vi "WeDo-PyBD.vi"() -> ()   [LabVIEW 2016]
uses:
  VIs/uPythonX/uPythonX.xctl
panel:
  in  "Tab Control":T1(tab)=enum."Line Follow"
  in  "WeDo Sniffing Code":T2(xcontrol)={"VISA Refnum in"="ASRL23::INSTR", "Python Code"="import machine, utime\n\nuart = machine.UART(3)\nuart.init(baudrate=2400, bits=8, parity=None, stop=1)\n\nutime.sleep_ms(1000)\n\nstring = ''\nsize = 1\nwhile True:\n     print(uart.read(uart.any()))\n     utime.sleep_ms(300)\n     size = uart.any()\n\nstring"}
  in  "WeDo":T2(xcontrol)={"VISA Refnum in"="ASRL12::INSTR", "Python Code"="import machine, utime, gc\n\nuart = machine.UART(1)\n\ndef send_value(uart,data):\n     value = (data & 0xFF)\n     payload = bytes([0xC0, value, 0xFF ^ 0xC0 ^ value])\n     uart.write(payload)\n\ndef initLPF2(uart):\n     tx = machine.Pin('P1', machine.Pin.OUT)\n     rx = machine.Pin('P0', machine.Pin.IN)\n     tx.value(0)\n     utime.sleep_ms(500)\n     tx.value(1)\n     uart.init(baudrate=2400, bits=8, parity=None, stop=1)\n     uart.write(b'\\x00')\n     uart.write(b'\\x40\\x23\\x9C')\n     uart.write(b'\\x49\\x02\\x01\\xB5')\n     uart.write(b'\\x52\\x00\\xC2\\x01\\x00\\x6E')\n     uart.write(b'\\x5F\\x00\\x00\\x00\\x02\\x00\\x00\\x00\\x02\\xA0')\n     uart.write(b'\\x9A\\x00\\x4C\\x50\\x46\\x32\\x2D\\x43\\x41\\x4C\\x6E')\n     uart.write(b'\\x9A\\x01\\x00\\x00\\x00\\x00\\x00\\xC0\\x7F\\x44\\x9F')\n     uart.write(b'\\x9A\\x02\\x00\\x00\\x00\\x00\\x00\\x00\\xC8\\x42\\xED')\n     uart.write(b'\\x9A\\x03\\x00\\x00\\x00\\x00\\x00\\xC0\\x7F\\x44\\x9D')\n     uart.write(b'\\x92\\x04\\x52\\x41\\x57\\x00\\x2D')\n     uart.write(b'\\x8A\\x05\\x10\\x00\\x60')\n     uart.write(b'\\x92\\x80\\x03\\x01\\x03\\x00\\xEC')\n     utime.sleep_ms(5)\n     print(uart.read(uart.any()))\n     uart.write(b'\\xA1\\x00\\x4C\\x50\\x46\\x32\\x2D\\x43\\x4F\\x55\\x4E\\x54\\x00\\x00\\x00\\x00\\x00\\x00\\x58')\n     uart.write(b'\\x99\\x01\\x00\\x00\\x00\\x00\\x00\\x00\\xC8\\x42\\xED')\n     uart.write(b'\\x99\\x02\\x00\\x00\\x00\\x00\\x00\\x00\\xC8\\x42\\xEE')\n     uart.write(b'\\x99\\x03\\x00\\x00\\x00\\x00\\x00\\x00\\xC8\\x42\\xEF')\n     uart.write(b'\\x91\\x04\\x43\\x4E\\x54\\x00\\x33')\n     uart.write(b'\\x89\\x05\\x10\\x00\\x63')\n     uart.write(b'\\x91\\x80\\x01\\x02\\x04\\x00\\xE9')\n     utime.sleep_ms(5)\n     print(uart.read(uart.any()))\n     uart.write(b'\\xA0\\x00\\x4C\\x50\\x46\\x32\\x2D\\x44\\x45\\x54\\x45\\x43\\x54\\x00\\x00\\x00\\x00\\x00\\x1D')\n     uart.write(b'\\x98\\x01\\x00\\x00\\x00\\x00\\x00\\x00\\x20\\x41\\x07')\n     uart.write(b'\\x98\\x02\\x00\\x00\\x00\\x00\\x00\\x00\\xC8\\x42\\xEF')\n     uart.write(b'\\x98\\x03\\x00\\x00\\x00\\x00\\x00\\x00\\x20\\x41\\x05')\n     uart.write(b'\\x80\\x04\\x00\\x7B')\n     uart.write(b'\\x88\\x05\\x10\\x00\\x62')\n     uart.write(b'\\x90\\x80\\x01\\x00\\x03\\x00\\xED')\n     utime.sleep_ms(5)\n     print(uart.read(uart.any()))\n     uart.write(b'\\x04')  \n     # wait for ACK\n     starttime = utime.time()\n     currenttime = starttime\n     while (currenttime-starttime) < 2000:\n          utime.sleep_ms(5)\n          data = uart.read(uart.any())\n          if data.find(b'\\x04') >= 0:\n               print('Success')\n               currenttime = starttime+3000   # stop the loop\n          else:\n               currenttime = utime.time()\n     # pull pin low\n     uart.deinit()\n     tx = machine.Pin('P1', machine.Pin.OUT)\n     tx.value(0)\n     utime.sleep_ms(10)\n     #change baudrate\n     uart.init(baudrate=115200, bits=8, parity=None, stop=1)\n\n# loop from -10 to 10\ni=0\ninitLPF2(uart)\nwhile True:\n     gc.collect()\n     send_value(uart,i)\n     i += 1\n     if i > 10: i=-10\n     utime.sleep_ms(200)\n"}
  in  "LPF2Class":T2(xcontrol)={"VISA Refnum in"="ASRL12::INSTR", "Python Code"="import machine, utime, gc\n\nfrom pyb import LED\n\nred_led   = LED(1)\ngreen_led = LED(2)\nblue_led  = LED(3)\nir_led    = LED(4)\n\nclass LPF2(object):\n     def __init__(self, uartChannel, txPin, rxPin):\n          self.txPin = txPin\n          self.rxPin = rxPin\n          self.uart = machine.UART(uartChannel)\n          self.connected = False\n\n     def send_value(self,data):\n          value = (data & 0xFF)\n          payload = bytes([0xC0, value, 0xFF ^ 0xC0 ^ value])\n          size = self.uart.write(payload)\n          if not size: self.connected = False\n\n     def initialize(self):\n          self.tx = machine.Pin(self.txPin, machine.Pin.OUT)\n          self.rx = machine.Pin(self.rxPin, machine.Pin.IN)\n          self.tx.value(0)\n          utime.sleep_ms(500)\n          self.tx.value(1)\n          self.uart.init(baudrate=2400, bits=8, parity=None, stop=1)\n          self.uart.write(b'\\x00')\n          self.uart.write(b'\\x40\\x23\\x9C')\n          self.uart.write(b'\\x49\\x02\\x01\\xB5')\n          self.uart.write(b'\\x52\\x00\\xC2\\x01\\x00\\x6E')\n          self.uart.write(b'\\x5F\\x00\\x00\\x00\\x02\\x00\\x00\\x00\\x02\\xA0')\n          self.uart.write(b'\\x9A\\x00\\x4C\\x50\\x46\\x32\\x2D\\x43\\x41\\x4C\\x6E')\n          self.uart.write(b'\\x9A\\x01\\x00\\x00\\x00\\x00\\x00\\xC0\\x7F\\x44\\x9F')\n          self.uart.write(b'\\x9A\\x02\\x00\\x00\\x00\\x00\\x00\\x00\\xC8\\x42\\xED')\n          self.uart.write(b'\\x9A\\x03\\x00\\x00\\x00\\x00\\x00\\xC0\\x7F\\x44\\x9D')\n          self.uart.write(b'\\x92\\x04\\x52\\x41\\x57\\x00\\x2D')\n          self.uart.write(b'\\x8A\\x05\\x10\\x00\\x60')\n          self.uart.write(b'\\x92\\x80\\x03\\x01\\x03\\x00\\xEC')\n          utime.sleep_ms(5)\n          #  print(uart.read(uart.any()))\n          self.uart.write(b'\\xA1\\x00\\x4C\\x50\\x46\\x32\\x2D\\x43\\x4F\\x55\\x4E\\x54\\x00\\x00\\x00\\x00\\x00\\x00\\x58')\n          self.uart.write(b'\\x99\\x01\\x00\\x00\\x00\\x00\\x00\\x00\\xC8\\x42\\xED')\n          self.uart.write(b'\\x99\\x02\\x00\\x00\\x00\\x00\\x00\\x00\\xC8\\x42\\xEE')\n          self.uart.write(b'\\x99\\x03\\x00\\x00\\x00\\x00\\x00\\x00\\xC8\\x42\\xEF')\n          self.uart.write(b'\\x91\\x04\\x43\\x4E\\x54\\x00\\x33')\n          self.uart.write(b'\\x89\\x05\\x10\\x00\\x63')\n          self.uart.write(b'\\x91\\x80\\x01\\x02\\x04\\x00\\xE9')\n          utime.sleep_ms(5)\n          # print(uart.read(uart.any()))\n          self.uart.write(b'\\xA0\\x00\\x4C\\x50\\x46\\x32\\x2D\\x44\\x45\\x54\\x45\\x43\\x54\\x00\\x00\\x00\\x00\\x00\\x1D')\n          self.uart.write(b'\\x98\\x01\\x00\\x00\\x00\\x00\\x00\\x00\\x20\\x41\\x07')\n          self.uart.write(b'\\x98\\x02\\x00\\x00\\x00\\x00\\x00\\x00\\xC8\\x42\\xEF')\n          self.uart.write(b'\\x98\\x03\\x00\\x00\\x00\\x00\\x00\\x00\\x20\\x41\\x05')\n          self.uart.write(b'\\x80\\x04\\x00\\x7B')\n          self.uart.write(b'\\x88\\x05\\x10\\x00\\x62')\n          self.uart.write(b'\\x90\\x80\\x01\\x00\\x03\\x00\\xED')\n          utime.sleep_ms(5)\n          # print(uart.read(uart.any()))\n          self.uart.write(b'\\x04')  \n          # wait for ACK\n          starttime = utime.time()\n          currenttime = starttime\n          while (currenttime-starttime) < 2000:\n               utime.sleep_ms(5)\n               data = self.uart.read(self.uart.any())\n               if data.find(b'\\x04') >= 0:\n                    self.connected = True\n                    currenttime = starttime+3000   # stop the loop\n               else:\n                    currenttime = utime.time()\n          # pull pin low\n          self.uart.deinit()\n          self.tx = machine.Pin(self.txPin, machine.Pin.OUT)\n          self.tx.value(0)\n          utime.sleep_ms(10)\n          #change baudrate\n          self.uart.init(baudrate=115200, bits=8, parity=None, stop=1)"}
  in  "ToSpike":T2(xcontrol)={"VISA Refnum in"="ASRL12::INSTR", "Python Code"="import LPF2Class\n\n# loop from -10 to 10\ni=0\nred_led.on()\nlpf2 = LPF2Class.LPF2(1, 'P1', 'P0')    # OpenMV\nlpf2.initialize()\n\nwhile True:\n     if not lpf2.connected:\n          red_led.on()\n          utime.sleep(1)\n          lpf2.initialize()\n     else:\n          red_led.off()\n          while lpf2.connected:\n               gc.collect()\n               lpf2.send_value(i)\n               i += 1\n               # print(lpf2.connected)\n               if i > 10: i=-10\n               utime.sleep_ms(200)\n"}
  in  "ToSpike 2":T2(xcontrol)={"VISA Refnum in"="ASRL12::INSTR", "Python Code"="import LPF2Class\nimport sensor, image, time\n\nenable_lens_corr = False # turn on for straighter lines...\n\nsensor.reset()\nsensor.set_pixformat(sensor.RGB565) # grayscale is faster\nsensor.set_framesize(sensor.QQVGA)\nsensor.skip_frames(time = 2000)\n\nmin_degree = 0\nmax_degree = 179\n\n\nred_led.on()\nlpf2 = LPF2Class.LPF2(1, 'P1', 'P0')    # OpenMV\nlpf2.connected = True\n#lpf2.initialize()\n\nwhile True:\n     img = sensor.snapshot()\n     if enable_lens_corr: img.lens_corr(1.8) # for 2.8mm lens...\n          \n     if not lpf2.connected:\n          red_led.on()\n          utime.sleep(1)\n          lpf2.initialize()\n     else:\n          red_led.off()\n          while lpf2.connected:\n               gc.collect()\n               rawLines = img.find_lines(threshold = 1000, theta_margin = 25, rho_margin = 25)\n               averageAngle = 0\n               for line in rawLines:\n                    if (min_degree <= line.theta()) and (line.theta() <= max_degree):\n                         img.draw_line(line.line(), color = (255, 0, 0))\n                         averageAngle + = line.theta()\n               value = averageAngle / len(rawLines)\n\n               lpf2.send_value(value)\n               print(value)\n               utime.sleep_ms(200)\n"}
  in  "Spike":T2(xcontrol)={"VISA Refnum in"="ASRL73::INSTR", "Python Code"="import hub,utime\n\nhub.port.B.info()\n\n# if info comes back with None - then you have to restart the pybaord\n\nwhile True:\n     try:\n          value = hub.port.B.device.get()[0]\n          # print(value)\n          hub.display.show(str(value))\n          utime.sleep(0.2)\n     except:\n          utime.sleep(1)\n"}
  in  "WeDo 2":T2(xcontrol)={"VISA Refnum in"="ASRL23::INSTR", "Python Code"="import machine, utime, gc\n\ndef send_value(data):\n     value = (data & 0xFF)\n     payload = bytes([0xC0, value, 0xFF ^ 0xC0 ^ value])\n     uart.write(payload)\n\nimport machine, network, ubinascii, ujson, urequests\n\nWiFi = network.WLAN()\n\nmac = ubinascii.hexlify(network.WLAN().config(\"mac\"),\":\").decode()\nprint(\"MAC address: \" + mac)\n\ndef connect():\n     EN1 = machine.Pin(\"W23\", machine.Pin.OUT, value=1)  # set power high for USB power (500mA now allowed)\n     if not WiFi.isconnected():\n          print (\"Connecting ..\")\n          WiFi.active(True)\n          WiFi.connect(\"Chris's iPhone\",\"00lly4r4uryu\")\n          i=0\n          while i < 25 and not WiFi.isconnected():\n               utime.sleep_ms(200)\n               i=i+1\n          if WiFi.isconnected():\n               print (\"Connection succeeded\")\n          else:\n               print (\"Connection failed\")     \n\nconnect()\nprint (\"WiFi: \",WiFi.isconnected())\n\n# Info\nTag = \"admin.HiPeaks.temperature\"\nType = \"DOUBLE\"\nValue = \"0\"\nKey = \"0MasdJmBFsHePZqAtGn-_3xky4M8rxeNPjaSO4H5u9\"\n\nurlBase = \"https://api.systemlinkcloud.com/nitag/v2/tags/\"\nheaders = {\"Accept\":\"application/json\",\"x-ni-api-key\":Key}\n\nurlValue = urlBase + Tag + \"/values/current\"\n\ndef grab_value():\n#     value = {'value':'0'}\n     try:\n          value = urequests.get(urlValue,headers=headers).text\n     except:\n          pass\n\n     data = ujson.loads(value)\n     result = data.get(\"value\").get(\"value\")\n     return result\n\n# prepare WeDo\n\ntx = machine.Pin('Y9', machine.Pin.OUT)\nrx = machine.Pin('Y10', machine.Pin.IN)\ntx.value(0)\nutime.sleep_ms(500)\ntx.value(1)\n\nuart = machine.UART(3)\nuart.init(baudrate=2400, bits=8, parity=None, stop=1)\n\nuart.write(b'\\x00')\nuart.write(b'\\x40\\x23\\x9C')\nuart.write(b'\\x49\\x02\\x01\\xB5')\nuart.write(b'\\x52\\x00\\xC2\\x01\\x00\\x6E')\nuart.write(b'\\x5F\\x00\\x00\\x00\\x02\\x00\\x00\\x00\\x02\\xA0')\nuart.write(b'\\x9A\\x00\\x4C\\x50\\x46\\x32\\x2D\\x43\\x41\\x4C\\x6E')\nuart.write(b'\\x9A\\x01\\x00\\x00\\x00\\x00\\x00\\xC0\\x7F\\x44\\x9F')\nuart.write(b'\\x9A\\x02\\x00\\x00\\x00\\x00\\x00\\x00\\xC8\\x42\\xED')\nuart.write(b'\\x9A\\x03\\x00\\x00\\x00\\x00\\x00\\xC0\\x7F\\x44\\x9D')\nuart.write(b'\\x92\\x04\\x52\\x41\\x57\\x00\\x2D')\nuart.write(b'\\x8A\\x05\\x10\\x00\\x60')\nuart.write(b'\\x92\\x80\\x03\\x01\\x03\\x00\\xEC')\nutime.sleep_ms(5)\nprint(uart.read(uart.any()))\nuart.write(b'\\xA1\\x00\\x4C\\x50\\x46\\x32\\x2D\\x43\\x4F\\x55\\x4E\\x54\\x00\\x00\\x00\\x00\\x00\\x00\\x58')\nuart.write(b'\\x99\\x01\\x00\\x00\\x00\\x00\\x00\\x00\\xC8\\x42\\xED')\nuart.write(b'\\x99\\x02\\x00\\x00\\x00\\x00\\x00\\x00\\xC8\\x42\\xEE')\nuart.write(b'\\x99\\x03\\x00\\x00\\x00\\x00\\x00\\x00\\xC8\\x42\\xEF')\nuart.write(b'\\x91\\x04\\x43\\x4E\\x54\\x00\\x33')\nuart.write(b'\\x89\\x05\\x10\\x00\\x63')\nuart.write(b'\\x91\\x80\\x01\\x02\\x04\\x00\\xE9')\nutime.sleep_ms(5)\nprint(uart.read(uart.any()))\nuart.write(b'\\xA0\\x00\\x4C\\x50\\x46\\x32\\x2D\\x44\\x45\\x54\\x45\\x43\\x54\\x00\\x00\\x00\\x00\\x00\\x1D')\nuart.write(b'\\x98\\x01\\x00\\x00\\x00\\x00\\x00\\x00\\x20\\x41\\x07')\nuart.write(b'\\x98\\x02\\x00\\x00\\x00\\x00\\x00\\x00\\xC8\\x42\\xEF')\nuart.write(b'\\x98\\x03\\x00\\x00\\x00\\x00\\x00\\x00\\x20\\x41\\x05')\nuart.write(b'\\x80\\x04\\x00\\x7B')\nuart.write(b'\\x88\\x05\\x10\\x00\\x62')\nuart.write(b'\\x90\\x80\\x01\\x00\\x03\\x00\\xED')\nutime.sleep_ms(5)\nprint(uart.read(uart.any()))\nuart.write(b'\\x04')\n\n# wait for ACK\nstarttime = utime.time()\ncurrenttime = starttime\n\nwhile (currenttime-starttime) < 2000:\n     utime.sleep_ms(5)\n     data = uart.read(uart.any())\n     if data.find(b'\\x04') >= 0:\n          print('Success')\n          currenttime = starttime+3000   # stop the loop\n     else:\n          currenttime = utime.time()\n\n# pull pin low\nuart.deinit()\ntx = machine.Pin('Y9', machine.Pin.OUT)\ntx.value(0)\nutime.sleep_ms(10)\n\n#change baudrate\n\nuart.init(baudrate=115200, bits=8, parity=None, stop=1)\n\n# loop from -10 to 10\ni=0\n\nwhile True:\n     gc.collect()\n     data = grab_value()\n     send_value(data)\n     i += 1\n     if i > 10: i=-10\n     utime.sleep_ms(200)\n"}
  in  "Test":T2(xcontrol)={"VISA Refnum in"="ASRL23::INSTR", "Python Code"="import machine, utime\n\n\nuart = machine.UART(6)\nuart.init(baudrate=2400, bits=8, parity=None, stop=1)\n\nuart.write(b'\\x40\\x23\\x9C')\nutime.sleep_ms(1000)\nuart.read(uart.any())"}
  in  "Hub":T2(xcontrol)={"VISA Refnum in"="ASRL24::INSTR", "Python Code"="import hub,utime\n\n# no idea how to read a sesnor value on flipper - how do I read the \n#accelerometer as well?\n\nhub.button.left.is_pressed()\n\nhub.button.left.presses()\n\nhub.button.left.was_pressed()\n\nhub.port.A.device.get(0)\n\nwhile True:\n     hub.port.A.device.get(2)\n     utime.sleep_ms(200)"}
  in  "OLED display":T2(xcontrol)={"VISA Refnum in"="ASRL24::INSTR", "Python Code"="# https://learn.adafruit.com/adafruit-oled-featherwing/python-circuitpython-wiring\n\n# 128 x 32 monochrome - i2c address 0x3C\n\nimport pyb,utime\n#import adafruit_ssd1306\n\nSET_CONTRAST        = 0x81\nSET_ENTIRE_ON       = 0xa4\nSET_NORM_INV        = 0xa6\nSET_DISP            = 0xae\nSET_MEM_ADDR        = 0x20\nSET_COL_ADDR        = 0x21\nSET_PAGE_ADDR       = 0x22\nSET_DISP_START_LINE = 0x40\nSET_SEG_REMAP       = 0xa0\nSET_MUX_RATIO       = 0xa8\nSET_COM_OUT_DIR     = 0xc0\nSET_DISP_OFFSET     = 0xd3\nSET_COM_PIN_CFG     = 0xda\nSET_DISP_CLK_DIV    = 0xd5\nSET_PRECHARGE       = 0xd9\nSET_VCOM_DESEL      = 0xdb\nSET_CHARGE_PUMP     = 0x8d\n\naddr=0x3c\nheight = 32\nwidth = 128\npages = height // 8\nbuffer = bytearray ((pages * width) + 1)\nbuffer[0] = 0x40\n\ni2c = machine.I2C(2)\n#i2c.scan()\n#should see a 60\n\n\n\ndef write_cmd(cmd):\n     \n     temp = bytearray(2)\n     temp[0] = 0x80 # Co=1, D/C#=0\n     temp[1] = cmd\n     i2c.writeto(addr,temp)\n\ndef poweron():\n     \"Reset device and turn on the display.\"\n     RST.value(1)\n     utime.sleep_ms(1)\n     RST.value(0)\n     utime.sleep_ms(10)\n     RST.value(1)\n     utime.sleep_ms(10)\n     write_cmd(SET_DISP | 0x01)\n     \ndef init_display():\n     \" initilaize display \"\n     write_cmd(SET_DISP | 0x00) # turn off\n     write_cmd(SET_MEM_ADDR, 0x00)  # horizontal\n     write_cmd(SET_DISP_START_LINE | 0x00)  # \n     write_cmd(SET_SEG_REMAP | 0x01) # col addr 127 maped to SEG0\n     write_cmd(SET_MUX_RATIO)\n     write_cmd(height - 1)\n     write_cmd(SET_COM_OUT_DIR | 0x08)\n     write_cmd(SET_DISP_OFFSET, 0x00)\n     write_cmd(SET_COM_PIN_CFG, 0x02 if self.height == 32 else 0x12)\n     write_cmd(SET_DISP_CLK_DIV, 0x80)\n     write_cmd(SET_PRECHARGE, 0x22 if self.external_vcc else 0xf1)\n     write_cmd(SET_VCOM_DESEL, 0x30)\n     write_cmd(SET_CONTRAST, 0xff)\n     write_cmd(SET_ENTIRE_ON)\n     write_cmd(SET_NORM_INV)\n     write_cmd(SET_CHARGE_PUMP, 0x10 if self.external_vcc else 0x14)\n     write_cmd(SET_DISP | 0x01)\n     show()\n     \ndef show():\n     \"update display\"\n     xpos0 = 0\n     xpos1 = width - 1\n     if width == 64:\n            # displays with width of 64 pixels are shifted by 32\n            xpos0 += 32\n            xpos1 += 32\n     write_cmd(SET_COL_ADDR)\n     write_cmd(xpos0)\n     write_cmd(xpos1)\n     write_cmd(SET_PAGE_ADDR)\n     write_cmd(0)\n     write_cmd(pages - 1)\n     write_framebuf()\n\ndef write_framebuf():\n     i2c.writeto(addr,buffer)\n\ndef poweroff():\n        \"\"\"Turn off the display (nothing visible)\"\"\"\n     write_cmd(SET_DISP | 0x00)\n\ndef contrast(contrast):\n        \"\"\"Adjust the contrast\"\"\"\n     write_cmd(SET_CONTRAST)\n     write_cmd(contrast)\n\ndef invert(invert):\n        \"\"\"Invert all pixels on the display\"\"\"\n     write_cmd(SET_NORM_INV | (invert & 1))\n\n# W16, 22, 24\nA = pyb.Pin('W24', pyb.Pin.IN, pull=pyb.Pin.PULL_UP)\nB = pyb.Pin('W22', pyb.Pin.IN, pull=pyb.Pin.PULL_UP)\nC = pyb.Pin('W16', pyb.Pin.IN, pull=pyb.Pin.PULL_UP)\nRST =  pyb.Pin('W29', pyb.Pin.IN, pull=pyb.Pin.PULL_UP)\n\npoweron()\n\nwhile True:\n#     print(str(A.value()) + ' ' + str(B.value()) + ' ' + str(C.value()))\n     i2c.readfrom(addr)\n     utime.sleep_ms(100)\n     \n\n"}
  # "https://www.sparkfun.com/qwiic"
  # ">>> uart.read(uart.any())\nb'\\x00\\x00\\x00\\x00\\x00\\x00R\\x00\\xc2\\x01\\x00n\\x04\\xff'"
  # "Blue"
  # "Green"
  # "Yellow"
  # "Red"
  # "Orange"
  # "Magenta"
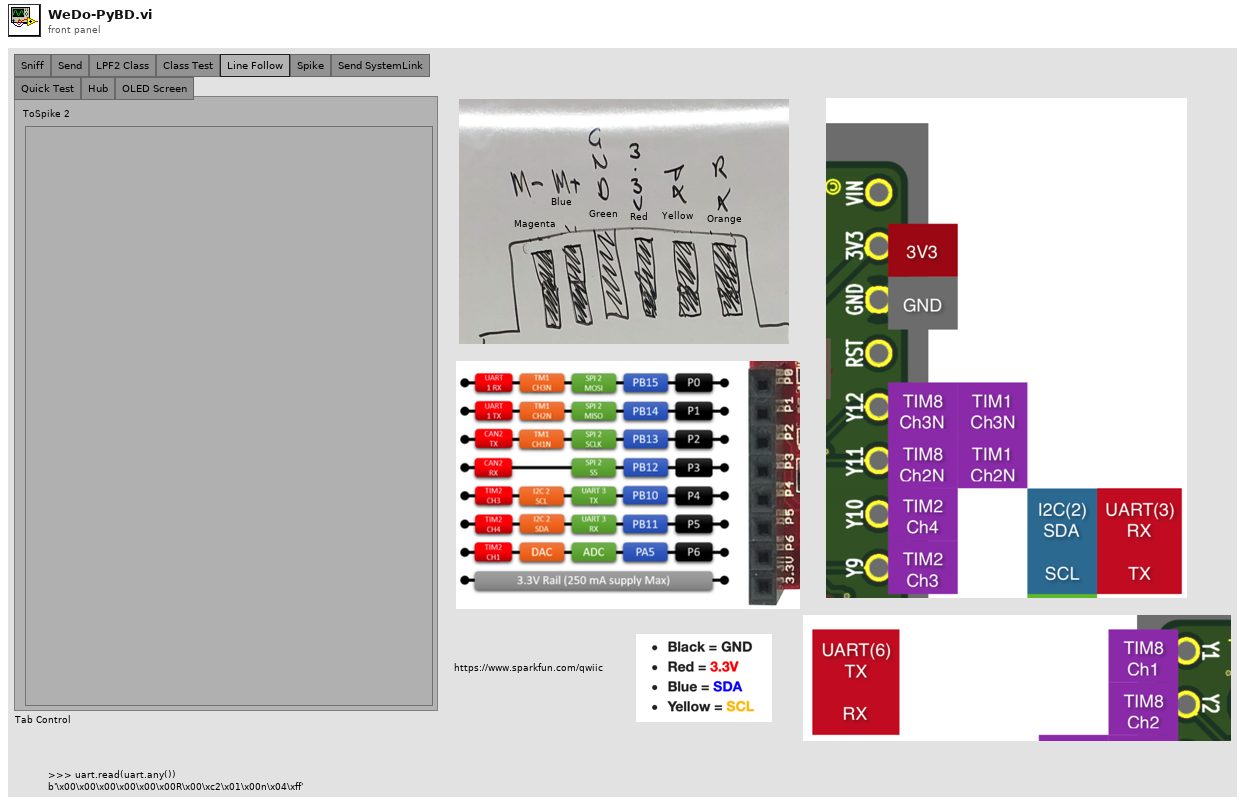
[diagram p1: front panel]
types:
  T1 = enum32{"Sniff", "Send", "LPF2 Class", "Class Test", "Line Follow", "Spike", "Send SystemLink", "Quick Test", "Hub", "OLED Screen"}
  T2 = cluster{"VISA Refnum in":refnum<visa-resource-name>, "Python Code":string}
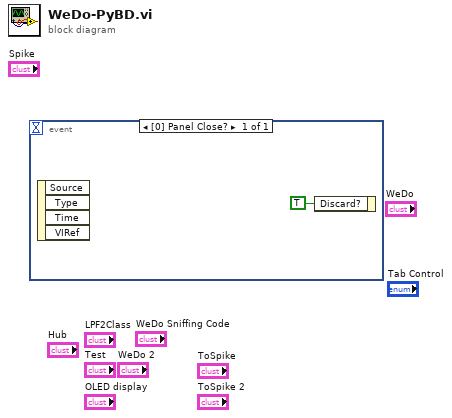
[diagram p0: block diagram]
diagram:
  n1 = event shown="[0] Panel Close?" {
    selector: _ -> [_]
    dyn-events: _ -> [_]
    timeout: _ -> [_]
    event Panel Close? {
      n2 = event-data() -> ()  [unwired: 1 in, 4 out]
      n3 = event-data("Discard?"=TRUE) -> ()  [unwired: 1 in, 1 out]
    }
  }
